vi "Connect to IP Address.vi"(8 "error in (no error)":errorcluster, 11 "Device Ref in":T1 format="%.0x") -> (0 "error out":errorcluster, 2 "REST Client out":refnum<class "REST Client.lvclass">, 3 "Item Ref out":T1 format="%.0x")   [LabVIEW 2020, in "G5 Regatron Custom Device Engine.lvlib"]
uses:
  G5 Regatron Custom Device Engine.lvlib
  <vilib>/NI VeriStand/Custom Device API/Custom Device Item Ref.ctl
  <vilib>/addons/_JKI.lib/REST Client/classes/REST Client/REST Client.lvclass
  Shared/Constants.vi
  <vilib>/NI VeriStand/Custom Device API/Get Item Property (String).vi
  <vilib>/NI VeriStand/Custom Device API/Custom Device API.lvlib
  Shared/Regatron.G5.Rest.lvlib
  Shared/G5 Regatron Custom Device Shared.lvlib
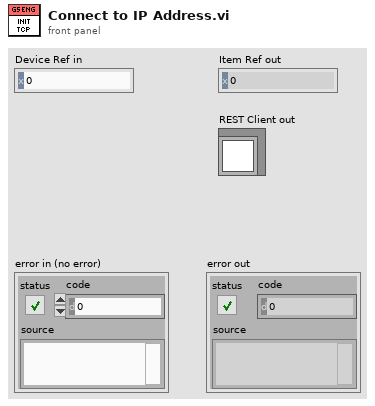
[diagram p1: front panel]
types:
  T1 = typedef "Custom Device API.lvlib/Custom Device Item Ref.ctl" = u64
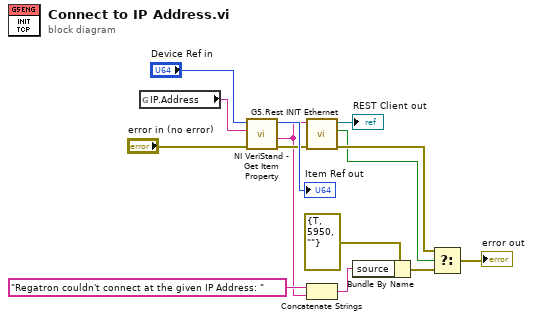
[diagram p0: block diagram]
diagram:
  n1 = global read "Constants.vi" "IP.Address"() -> (w2:string)
  n2 = call-poly <vilib>:"NI VeriStand - Get Item Property.vi"("error in (no error)"="error in (no error)", "Property Name"=w2, "Item Ref in"="Device Ref in") -> ("error out"=w10:errorcluster, "Value"=w3:string, "Item Ref out"=→"Item Ref out":T1)  [unwired: 5 in, 1 out]
  n3 = call "G5.Rest INIT Ethernet.vi"("error in (no error)"=w10, "IP"=w3) -> ("error out"=w9:errorcluster, "Device found"=w8:bool, "G5 WEB API"=→"REST Client out":refnum<class "REST Client.lvclass">)  [unwired: 5 in, 2 out]
  n4 = Concatenate Strings("Regatron couldn't connect at the given IP Address: " ("source"), w3) -> (w4:string)
  n5 = Bundle By Name(cluster=errorcluster {"status"=TRUE, "code"=5950, "source"=""} ("f"), "source"=w4) -> (w6:errorcluster)
  n6 = Select(t=w9, s=w8, f=w6) -> (s? t:f=→"error out":errorcluster)
